vi "set_context.vi"(7 "context":string, 8 "error in (no error)":errorcluster, 11 "Queue Log Provider in":refnum<class "NIErrLog Log Provider.lvclass">) -> (0 "error out":errorcluster, 3 "Queue Log Provider out":refnum<class "NIErrLog Log Provider.lvclass">)   [LabVIEW 2019, in "LVCOOOP.lvlib" / "Support API.lvlib" / "NIErrLog Log Provider.lvclass"]
uses:
  NIErrLog Log Provider.lvclass
  NIErrLog Log Provider.lvclass/NIErrLog Log Provider.ctl
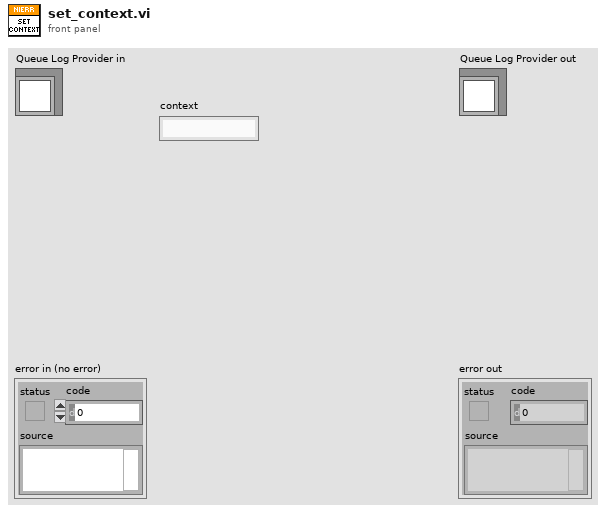
[diagram p1: front panel]
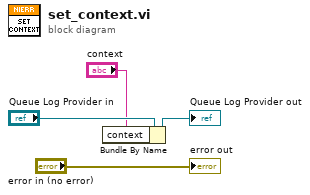
[diagram p0: block diagram]
diagram:
  n1 = Bundle By Name(cluster="Queue Log Provider in", "context"="context") -> (→"Queue Log Provider out":refnum<class "NIErrLog Log Provider.lvclass">)
  "error out" <- "error in (no error)"
